vi "Get Interactions.vi"(8 "error in (no error)":errorcluster, 11 "Topas4 in":refnum<class "Topas4.lvclass">) -> (0 "error out":errorcluster, 1 "Ranges":cluster{"Upper":dbl, "Lower":dbl}[](array[cluster]), 2 "Interaction Types":string[](array[string]), 3 "Topas4 out":refnum<class "Topas4.lvclass">)   [LabVIEW 2020, in "Topas4.lvclass"]
uses:
  Topas4.lvclass
  Topas4-LabVIEW-Driver/Library/Topas4.lvlib
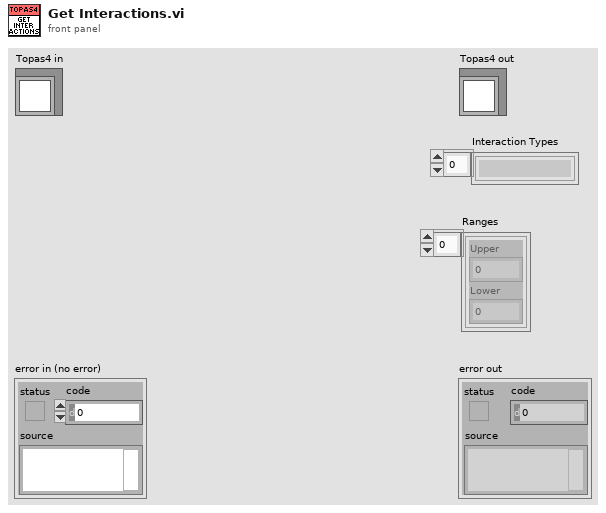
[diagram p1: front panel]
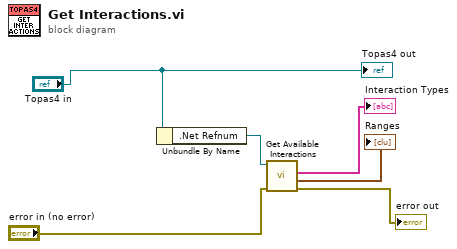
[diagram p0: block diagram]
diagram:
  n1 = Unbundle By Name("Topas4 in") -> (".Net Refnum"=w5:refnum<k24>)
  n2 = call "Get Available Interactions.vi"("error in"="error in (no error)", "reference"=w5) -> ("error out"=→"error out":errorcluster, "Interaction Ranges"=→"Ranges":cluster{"From":dbl, "To":dbl}[], "Interaction Types"=→"Interaction Types":string[])  [unwired: 6 in, 1 out]
  "Topas4 out" <- "Topas4 in"
